vi "Set Protocol-Specific Properties.vi"() -> ()   [LabVIEW 2019, in "Scripting API.lvlib"]
uses:
  Scripting API.lvlib
  niveristand-instrument-addon-classes/Source/Protocols/Protocol Parent/Types/Base Protocol Type.ctl
  niveristand-instrument-addon-classes/Source/Protections/Parent Protection/Protection.lvclass
  niveristand-instrument-addon-classes/Source/Protocols/Protocol Parent/Protocol Parent.lvclass
  <vilib>/regexp/Match Regular Expression.xnode
panel:
  out "Array 2":errorcluster[](array[cluster])
  out "Array 3":errorcluster[](array[cluster])
  out "array w/ subset deleted 2":string[](array[string])
  out "array w/ subset deleted":string[](array[string])
  out "Array":T1[](array[typedef])
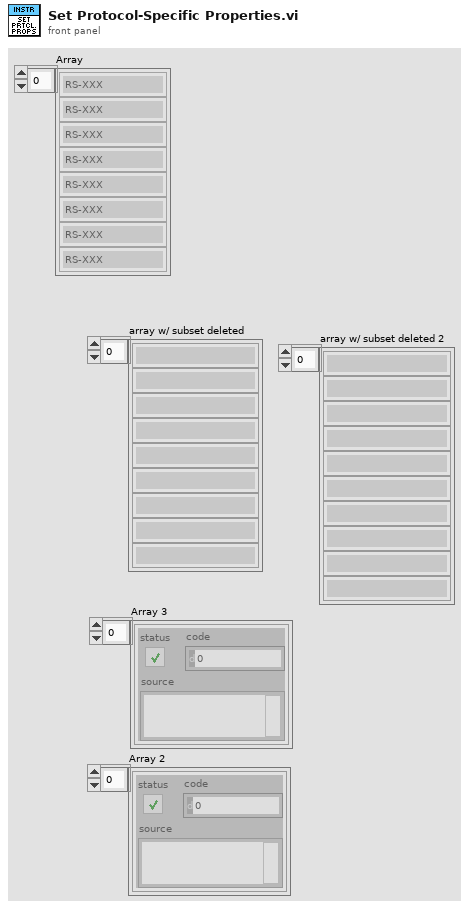
[diagram p1: front panel]
types:
  T1 = typedef "Protocols.lvlib/Protocol Parent.lvclass/Base Protocol Type.ctl" = enum16{"RS-XXX", "VISA", "TCPIP", "UDP", "GPIB ConvBox"}
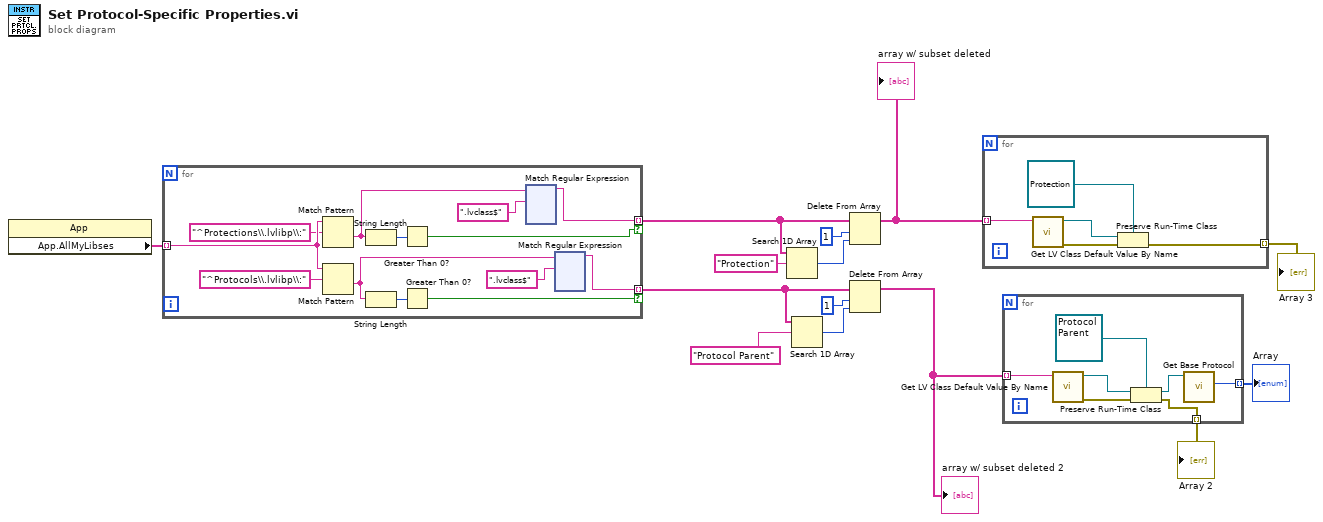
[diagram p0: block diagram]
diagram:
  n1 = property class="App"() -> ("App.AllMyLibses"=w14:string[])  [unwired: 2 in, 2 out]
  n2 = for {
    tunnel: w14 -> [w22] mode=indexing
    tunnel: [w17] -> w11 mode=indexing if=w26
    tunnel: [w19] -> w13 mode=indexing if=w24
    n3 = Match Pattern(string=w22, regular expression="^Protections\\.lvlibp\\:" ("search string/char (-)")) -> (after substring=w16:string)  [unwired: 1 in, 3 out]
    n4 = Match Pattern(string=w22, regular expression="^Protocols\\.lvlibp\\:" ("search string/char (-)")) -> (after substring=w15:string)  [unwired: 1 in, 3 out]
    n5 = String Length(string=w16) -> (length=w25:i32)
    n6 = String Length(string=w15) -> (length=w27:i32)
    n7 = Greater Than 0?(x=w25) -> (x > 0?=w24:bool)
    n8 = Greater Than 0?(x=w27) -> (x > 0?=w26:bool)
    n9 = xnode "Match Regular Expression"("input string"=w16, "regular expression"=".lvclass$") -> ("before match"=w19:string)  [unwired: 4 in, 4 out]
    n10 = xnode "Match Regular Expression"("input string"=w15, "regular expression"=".lvclass$") -> ("before match"=w17:string)  [unwired: 4 in, 4 out]
  }
  n11 = Search 1D Array(1D array=w13, element="Protection") -> (index of element=w7:i32)  [unwired: 1 in]
  n12 = Search 1D Array(1D array=w11, element="Protocol Parent") -> (index of element=w9:i32)  [unwired: 1 in]
  n13 = Delete From Array(array=w13, length=1, index=w7) -> (array with subset deleted=w12:string[])  [unwired: 1 out]
  "array w/ subset deleted" <- w12
  n14 = Delete From Array(array=w11, length=1, index=w9) -> (array with subset deleted=w10:string[])  [unwired: 1 out]
  "array w/ subset deleted 2" <- w10
  n15 = for {
    tunnel: w12 -> [w260] mode=indexing
    tunnel: [w256] -> w2 mode=indexing
    n16 = call <vilib>:"Get LV Class Default Value By Name.vi"("class name"=w260) -> ("error out"=w258:errorcluster, "object"=w259:refnum<class>)  [unwired: 9 in]
    n17 = Preserve Run-Time Class(object in=w259, error in=w258, 2:refnum<class "Protection.lvclass"> refnum ("Protections.lvlib:Protection.lvclass")) -> (error out=w256:errorcluster)  [unwired: 1 out]
  }
  "Array 3" <- w2
  n18 = for {
    tunnel: w10 -> [w267] mode=indexing
    tunnel: [w262] -> w3 mode=indexing
    tunnel: [w261] -> w1 mode=indexing
    n19 = call <vilib>:"Get LV Class Default Value By Name.vi"("class name"=w267) -> ("error out"=w264:errorcluster, "object"=w266:refnum<class>)  [unwired: 9 in]
    n20 = Preserve Run-Time Class(object in=w266, error in=w264, 2:refnum<class "Protocol Parent.lvclass"> refnum ("Protocols.lvlib:Protocol Parent.lvclass")) -> (object out=w263:refnum<class "Protocol Parent.lvclass">, error out=w261:errorcluster)
    n21 = call-dynamic "Get Base Protocol.vi"("Protocol Parent in"=w263) -> ("Protocol out"=w262:T1)  [unwired: 8 in, 2 out]
  }
  "Array" <- w3
  "Array 2" <- w1
